vi "DSP Configuration.vi"(8 "error in (no error)":errorcluster caption="错误输入（无错误）", 11 "DSP Parameter Input":T1={"Sampling Frequency"=0.0, "filter type"=enum."Lowpass", "RF Filter Low Frequency"=0.0, "RF Filter High Frequency"=0.0, "RF Filter Taps"=0, "window"=0, "RF window parameter"=nan, "filter type 2"=enum."Lowpass", "Demodulated Filter Low Frequency"=0.0, "Demodulated Filter HighFrequency"=0.0, "Demodulated Filter Order"=0, "SPAN"=0, "Logarithmic Base"=0.0, "Noise path"="", "Work position parameter"=[]} {"window" items=["Rectangle"=0, "Hanning"=1, "Hamming"=2, "Blackman-Harris"=3, "Exact Blackman"=4, "Blackman"=5, "Flat Top"=6, "4 Term B-Harris "=7, "7 Term B-Harris"=8, "Low Sidelobe"=9, "Blackman Nuttall"=11, "Triangle"=30, "Bartlett-Hanning"=31, "Bohman"=32, "Parzen"=33, "Welch"=34, "Kaiser"=60, "Dolph-Chebyshev"=61, "Gaussian"=62]}) -> (0 "error out":errorcluster caption="错误输出", 3 "DSP Parameter Output":T1={"Sampling Frequency"=0.0, "filter type"=enum."Lowpass", "RF Filter Low Frequency"=0.0, "RF Filter High Frequency"=0.0, "RF Filter Taps"=0, "window"=0, "RF window parameter"=nan, "filter type 2"=enum."Lowpass", "Demodulated Filter Low Frequency"=0.0, "Demodulated Filter HighFrequency"=0.0, "Demodulated Filter Order"=0, "SPAN"=0, "Logarithmic Base"=0.0, "Noise path"="", "Work position parameter"=[]} {"window" items=["Rectangle"=0, "Hanning"=1, "Hamming"=2, "Blackman-Harris"=3, "Exact Blackman"=4, "Blackman"=5, "Flat Top"=6, "4 Term B-Harris "=7, "7 Term B-Harris"=8, "Low Sidelobe"=9, "Blackman Nuttall"=11, "Triangle"=30, "Bartlett-Hanning"=31, "Bohman"=32, "Parzen"=33, "Welch"=34, "Kaiser"=60, "Dolph-Chebyshev"=61, "Gaussian"=62]})   [LabVIEW 2015, in "Digital Signal Processing.lvlib"]
doc: "该模板用于创建子VI。"
uses:
  Digital Signal Processing.lvlib
  Support/DSP Configuration.ctl
  <vilib>/Analysis/3filter.llb/Filter Passband Type.ctl
  <vilib>/Analysis/4window.llb/windowTd.ctl
  Utility VIs/Utility VIs.lvlib
  <vilib>/Analysis/NI_AALBase.lvlib
  <vilib>/Analysis/NI_AALPro.lvlib
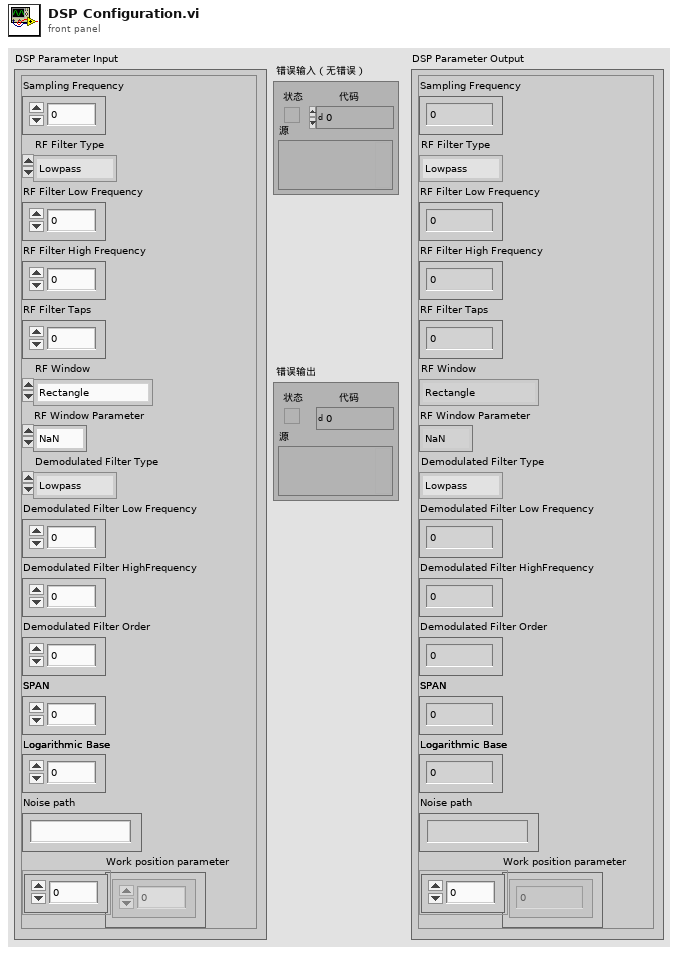
[diagram p1: front panel]
types:
  T1 = typedef "Digital Signal Processing.lvlib/DSP Configuration.ctl" = cluster{"Sampling Frequency":dbl, "filter type":T2, "RF Filter Low Frequency":dbl, "RF Filter High Frequency":dbl, "RF Filter Taps":i32, "window":T3, "RF window parameter":dbl, "filter type 2":T2, "Demodulated Filter Low Frequency":dbl, "Demodulated Filter HighFrequency":dbl, "Demodulated Filter Order":i32, "SPAN":i32, "Logarithmic Base":dbl, "Noise path":string, "Work position parameter":i32[]}
  T2 = typedef "NI_AALBase.lvlib/Filter Passband Type.ctl" = enum32{"Lowpass", "Highpass", "Bandpass", "Bandstop"}
  T3 = typedef "NI_AALPro.lvlib/windowTd.ctl" = u32
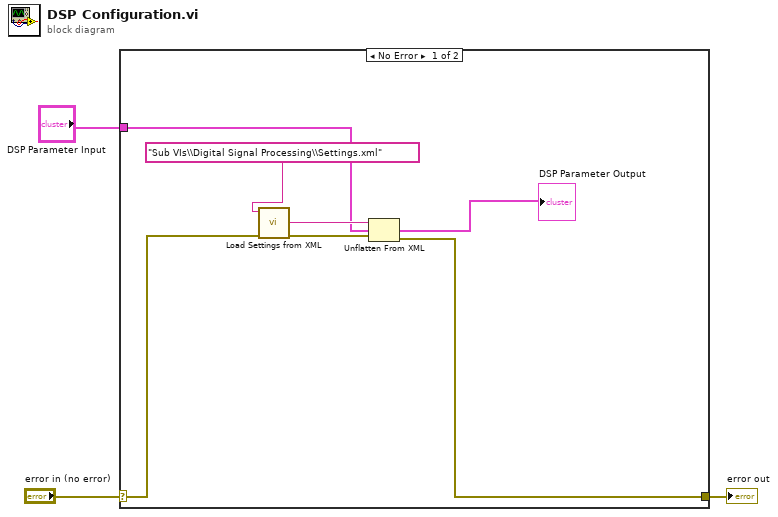
[diagram p0: block diagram]
diagram:
  n1 = case shown="No Error" "error in (no error)" {
    selector: "error in (no error)" -> [w6 w11]
    tunnel: [w5 w11] -> w2
    tunnel: "DSP Parameter Input" -> [w8 _]
    frame No Error {
      n2 = call "Load Settings from XML.vi"("error in (no error)"=w6, "名称或相对路径"="Sub VIs\\Digital Signal Processing\\Settings.xml") -> ("error out"=w7:errorcluster, "XML Elements"=w9:string)  [unwired: 8 in]
      n3 = Unflatten From XML(xml string=w9, type=w8, error in (no error)=w7) -> (value=→"DSP Parameter Output":T1, error out=w5:errorcluster)
    }
    frame Error {
    }
  }
  "error out" <- w2
